vi "Lift Cases.vi"() -> ()   [LabVIEW 2014]
uses:
  Begin/Global Variables.vi
  Begin/Global RefNums.vi
panel:
  in  "Tote 1 Height":dbl=7.0
  in  "Tote 3 Height":dbl=41.0
  in  "Lift Speed":dbl=0.75 format="%#_13g"
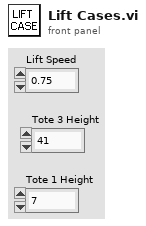
[diagram p1: front panel]
types:
  T1 = typedef "WPI_SwitchDevRef.ctl" = cluster{"DevStatus":errorcluster, "DIO Channel":T2, "Controller":T3, "CntIndex":T4, "Normally Closed":bool}
  T2 = typedef "FPGA_DIOChannel.ctl" = enum8{"DIO 0", "DIO 1", "DIO 2", "DIO 3", "DIO 4", "DIO 5", "DIO 6", "DIO 7", "DIO 8", "DIO 9", "DIO MXP 0", "DIO MXP 1", "DIO MXP 2", "DIO MXP 3", "DIO MXP 4", "DIO MXP 5", "DIO MXP 6", "DIO MXP 7", "DIO MXP 8", "DIO MXP 9", "DIO MXP 10", "DIO MXP 11", "DIO MXP 12", "DIO MXP 13", "DIO MXP 14", "DIO MXP 15", "Invalid"}
  T3 = typedef "FPGA_TypedefDigitalModule.ctl" = enum16{"Controller 1"}
  T4 = typedef "FPGA_CounterCtrSystemIndex.ctl" = enum8{"Ctr 0", "Ctr 1", "Ctr 2", "Ctr 3", "Ctr 4", "Ctr 5", "Ctr 6", "Ctr 7", "Invalid"}
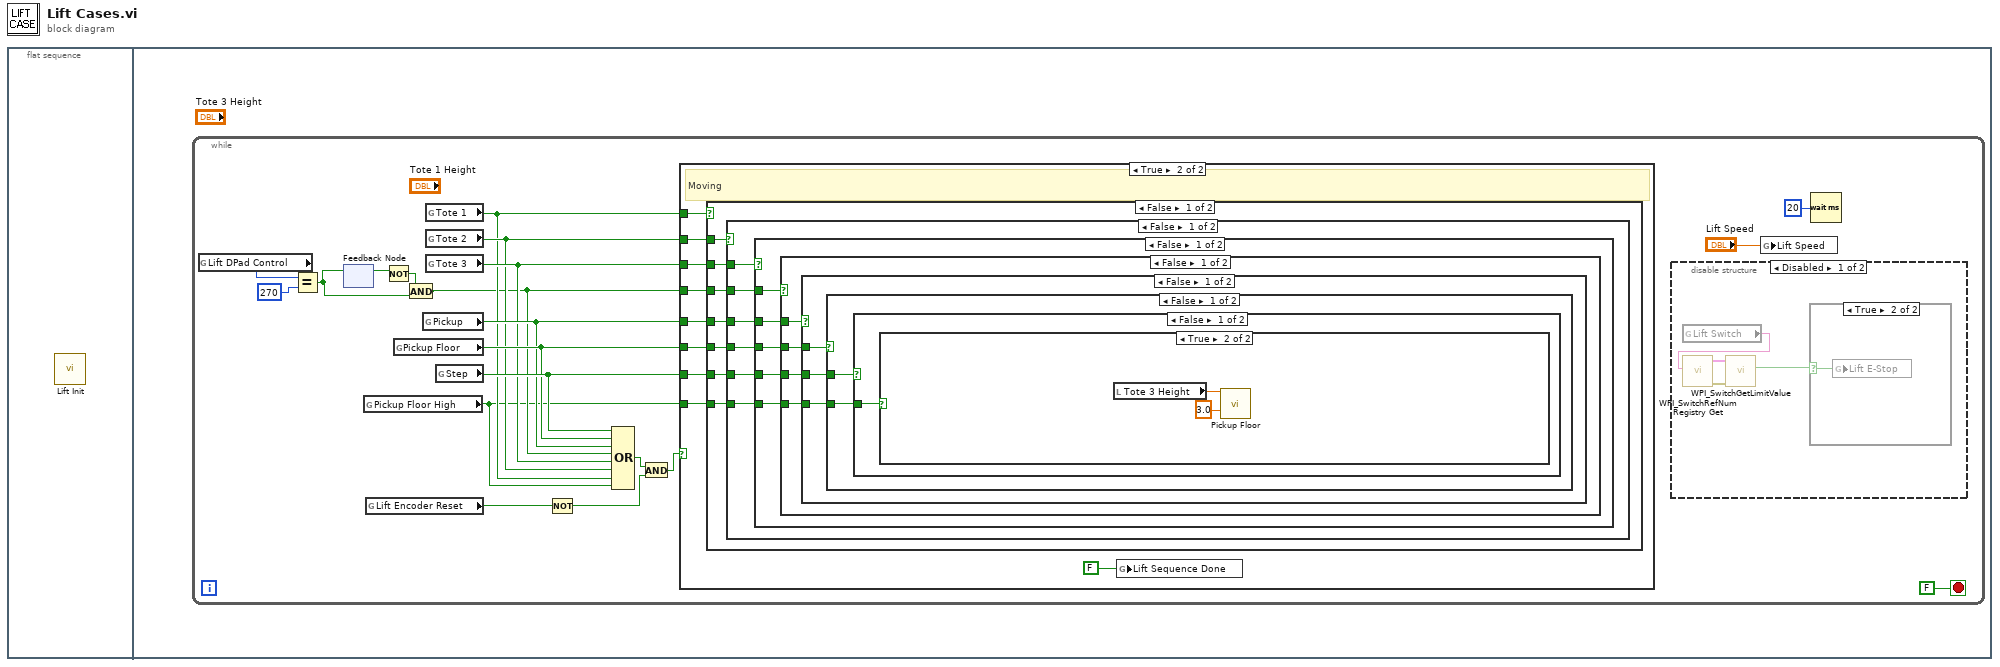
[diagram p0: block diagram]
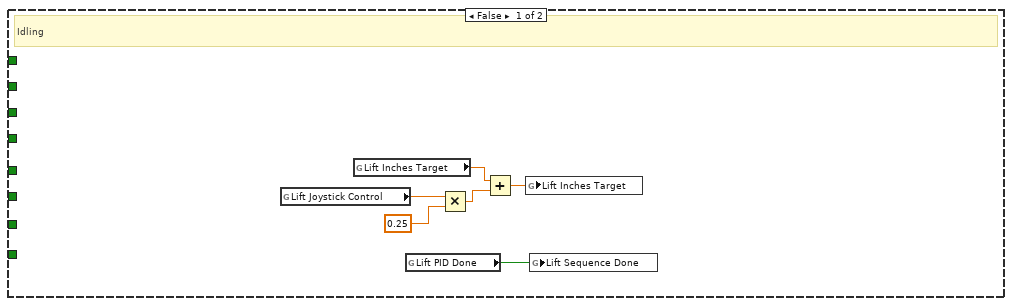
[diagram p4: hidden frame]
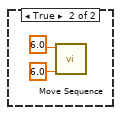
[diagram p6: hidden frame]
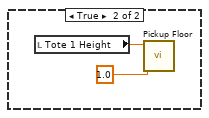
[diagram p7: hidden frame]
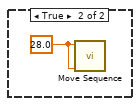
[diagram p8: hidden frame]
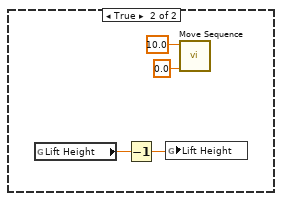
[diagram p9: hidden frame]
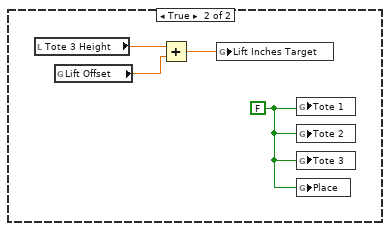
[diagram p10: hidden frame]
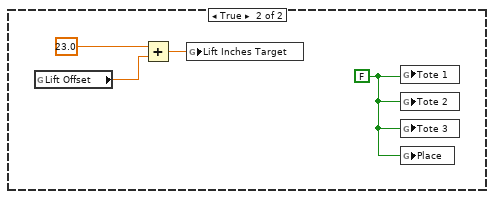
[diagram p11: hidden frame]
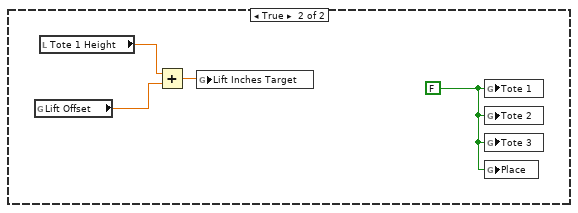
[diagram p12: hidden frame]
diagram:
  n1 = flat-sequence {
    frame #0 {
      n2 = call "Lift Init.vi"() -> ()  [unwired: 12 in]
    }
    frame #1 {
      n3 = while {
        stop <- FALSE stop-if-true
        n4 = global read "Global Variables.vi" "Lift DPad Control"() -> (w3:i16)
        n5 = Equal?(x=w3, y=i16 270) -> (x = y?=w8:bool)
        n6 = feedback #1() -> (w7:bool)  [unwired: 1 in]
        n7 = feedback-in #1(w8) -> ()
        n8 = global read "Global Variables.vi" "Pickup Floor High"() -> (w2:bool)
        n9 = global read "Global Variables.vi" "Lift Encoder Reset"() -> (w11:bool)
        n10 = Not(x=w7) -> (.not. x?=w6:bool)
        n11 = global read "Global Variables.vi" "Pickup Floor"() -> (w18:bool)
        n12 = And(x=w6, y=w8) -> (x .and. y?=w4:bool)
        n13 = global read "Global Variables.vi" "Pickup"() -> (w17:bool)
        n14 = global read "Global Variables.vi" "Tote 1"() -> (w14:bool)
        n15 = global read "Global Variables.vi" "Tote 2"() -> (w15:bool)
        n16 = global read "Global Variables.vi" "Tote 3"() -> (w16:bool)
        n17 = global read "Global Variables.vi" "Step"() -> (w19:bool)
        n18 = Not(x=w11) -> (.not. x?=w10:bool)
        n19 = Compound Arithmetic op=OR(w19, w18, w17, w4, w16, w15, w14, w2) -> (w12:bool)
        n20 = And(x=w12, y=w10) -> (x .and. y?=w9:bool)
        n21 = case shown="True" w9 {
          tunnel: w14 -> [_ w40]
          tunnel: w15 -> [_ w39]
          tunnel: w16 -> [_ w38]
          tunnel: w4 -> [_ w37]
          tunnel: w17 -> [_ w36]
          tunnel: w18 -> [_ w35]
          tunnel: w19 -> [_ w34]
          tunnel: w2 -> [_ w32]
          frame False {
            # "Idling"
            n22 = global read "Global Variables.vi" "Lift Joystick Control"() -> (w27:dbl)
            n23 = global read "Global Variables.vi" "Lift Inches Target"() -> (w29:dbl)
            n24 = global read "Global Variables.vi" "Lift PID Done"() -> (w31:bool)
            n25 = Multiply(x=w27, y=0.25) -> (x*y=w28:dbl)
            n26 = Add(x=w29, y=w28) -> (x+y=w30:dbl)
            n27 = global write "Global Variables.vi" "Lift Inches Target"(w30) -> ()
            n28 = global write "Global Variables.vi" "Lift Sequence Done"(w31) -> ()
          }
          frame True {
            # "Moving"
            n29 = case shown="False" w40 {
              tunnel: w39 -> [w47 _]
              tunnel: w38 -> [w46 _]
              tunnel: w37 -> [w45 _]
              tunnel: w36 -> [w44 _]
              tunnel: w35 -> [w43 _]
              tunnel: w34 -> [w42 _]
              tunnel: w32 -> [w41 _]
              frame False {
                n30 = case shown="False" w47 {
                  tunnel: w46 -> [w53 _]
                  tunnel: w45 -> [w52 _]
                  tunnel: w44 -> [w51 _]
                  tunnel: w43 -> [w50 _]
                  tunnel: w42 -> [w49 _]
                  tunnel: w41 -> [w48 _]
                  frame False {
                    n31 = case shown="False" w53 {
                      tunnel: w52 -> [w58 _]
                      tunnel: w51 -> [w57 _]
                      tunnel: w50 -> [w56 _]
                      tunnel: w49 -> [w55 _]
                      tunnel: w48 -> [w54 _]
                      frame False {
                        n32 = case shown="False" w58 {
                          tunnel: w57 -> [w62 _]
                          tunnel: w56 -> [w61 _]
                          tunnel: w55 -> [w60 _]
                          tunnel: w54 -> [w59 _]
                          frame False {
                            n33 = case shown="False" w62 {
                              tunnel: w61 -> [w65 _]
                              tunnel: w60 -> [w64 _]
                              tunnel: w59 -> [w63 _]
                              frame False {
                                n34 = case shown="False" w65 {
                                tunnel: w64 -> [w67 _]
                                tunnel: w63 -> [w66 _]
                                frame False {
                                n35 = case shown="False" w67 {
                                tunnel: w66 -> [w68 _]
                                frame False {
                                n36 = case shown="True" w68 {
                                frame False {
                                }
                                frame True {
                                n37 = local read "Tote 3 Height"() -> (w70:dbl)
                                n38 = call "Pickup Floor.vi"("Lift Height"=3.0, "Final Height"=w70) -> ()  [unwired: 10 in]
                                }
                                }
                                }
                                frame True {
                                n39 = call "Move Sequence.vi"("Distance Up"=6.0, "Distance Down"=6.0) -> ()  [unwired: 10 in]
                                }
                                }
                                }
                                frame True {
                                n40 = local read "Tote 1 Height"() -> (w74:dbl)
                                n41 = call "Pickup Floor.vi"("Lift Height"=1.0, "Final Height"=w74) -> ()  [unwired: 10 in]
                                }
                                }
                              }
                              frame True {
                                w75 = 28.0 ("Distance Down")
                                n42 = call "Move Sequence.vi"("Distance Up"=w75, "Distance Down"=w75) -> ()  [unwired: 10 in]
                              }
                            }
                          }
                          frame True {
                            n43 = global read "Global Variables.vi" "Lift Height"() -> (w77:dbl)
                            n44 = Decrement(x=w77) -> (x-1=w76:dbl)
                            n45 = global write "Global Variables.vi" "Lift Height"(w76) -> ()
                            n46 = call "Move Sequence.vi"("Distance Up"=0.0, "Distance Down"=10.0 ("Distance Down 2")) -> ()  [unwired: 10 in]
                          }
                        }
                      }
                      frame True {
                        w81 = FALSE ("Tote 0")
                        n47 = local read "Tote 3 Height"() -> (w80:dbl)
                        n48 = global read "Global Variables.vi" "Lift Offset"() -> (w82:dbl)
                        n49 = Add(x=w80, y=w82) -> (x+y=w83:dbl)
                        n50 = global write "Global Variables.vi" "Lift Inches Target"(w83) -> ()
                        n51 = global write "Global Variables.vi" "Tote 1"(w81) -> ()
                        n52 = global write "Global Variables.vi" "Tote 2"(w81) -> ()
                        n53 = global write "Global Variables.vi" "Tote 3"(w81) -> ()
                        n54 = global write "Global Variables.vi" "Place"(w81) -> ()
                      }
                    }
                  }
                  frame True {
                    w84 = FALSE ("Tote 0")
                    n55 = global read "Global Variables.vi" "Lift Offset"() -> (w85:dbl)
                    n56 = Add(x=23.0 ("x 2"), y=w85) -> (x+y=w86:dbl)
                    n57 = global write "Global Variables.vi" "Lift Inches Target"(w86) -> ()
                    n58 = global write "Global Variables.vi" "Tote 1"(w84) -> ()
                    n59 = global write "Global Variables.vi" "Tote 2"(w84) -> ()
                    n60 = global write "Global Variables.vi" "Tote 3"(w84) -> ()
                    n61 = global write "Global Variables.vi" "Place"(w84) -> ()
                  }
                }
              }
              frame True {
                w89 = FALSE ("Tote 0")
                n62 = global read "Global Variables.vi" "Lift Offset"() -> (w90:dbl)
                n63 = local read "Tote 1 Height"() -> (w88:dbl)
                n64 = Add(x=w88, y=w90) -> (x+y=w91:dbl)
                n65 = global write "Global Variables.vi" "Lift Inches Target"(w91) -> ()
                n66 = global write "Global Variables.vi" "Tote 1"(w89) -> ()
                n67 = global write "Global Variables.vi" "Tote 2"(w89) -> ()
                n68 = global write "Global Variables.vi" "Tote 3"(w89) -> ()
                n69 = global write "Global Variables.vi" "Place"(w89) -> ()
              }
            }
            n70 = global write "Global Variables.vi" "Lift Sequence Done"(FALSE ("Lift Sequence Done")) -> ()
          }
        }
        n71 = disable-structure shown="Disabled" {
          frame Disabled {
            n72 = global read "Global RefNums.vi" "Lift Switch"() -> (w22:string)
            n73 = call <vilib>:"WPI_SwitchRefNum Registry Get.vi"("refnum name"=w22) -> ("error out"=w24:errorcluster, "SwitchDevRef"=w23:T1)  [unwired: 9 in]
            n74 = call <vilib>:"WPI_SwitchGetLimitValue.vi"("error in (no error)"=w24, "SwitchDevRef"=w23) -> ("Switch Pressed"=w21:bool)  [unwired: 7 in, 2 out]
            n75 = case shown="True" w21 {
              selector: w21 -> [_ w25]
              frame False {
              }
              frame True {
                n76 = global write "Global Variables.vi" "Lift E-Stop"(w25) -> ()
              }
            }
          }
          frame Enabled {
          }
        }
        n77 = global write "Global Variables.vi" "Lift Speed"("Lift Speed") -> ()
        n78 = Wait (ms)(milliseconds to wait=u32 20) -> ()  [unwired: 1 out]
      }
    }
  }
